vi "Add.vi"(10 "DebugTracer":refnum<class "DebugTraceHandle.lvclass">, 11 "Name":string) -> ()   [LabVIEW 2024, in "DebugTraceSingleton.lvlib"]
uses:
  DebugTraceSingleton.lvlib
  DebugTraceHandle/DebugTraceHandle.lvclass
  Command.ctl
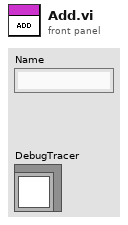
[diagram p1: front panel]
types:
  T1 = typedef "DebugTraceSingleton.lvlib/Command.ctl" = enum16{"Add", "Remove", "Get", "GetAll"}
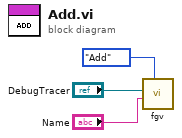
[diagram p0: block diagram]
diagram:
  n1 = call "fgv.vi"("Command"=Command."Add", "Name"="Name", "DebugTracer"="DebugTracer") -> ()  [unwired: 6 in, 3 out]
